vi "DM check burst group.vi"(11 "group":string) -> (3 "String":string)   [LabVIEW 2019, in "DataManagment.lvlib"]
uses:
  DataManagment.lvlib
  SubVIs/Shared/System GV.vi
  SubVIs/Shared/Shared.lvlib
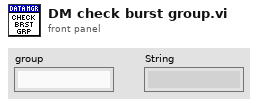
[diagram p1: front panel]
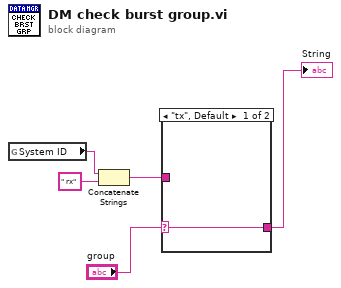
[diagram p0: block diagram]
diagram:
  n1 = global read "System GV.vi" "System ID"() -> (w1:string)
  n2 = Concatenate Strings(w1, " rx" ("group")) -> (w4:string)
  n3 = case shown="\"tx\", Default" "group" {
    selector: "group" -> [w6 _]
    tunnel: w4 -> [_ w7]
    tunnel: [w6 w7] -> w5
    frame "tx", Default {
    }
    frame "rx" {
    }
  }
  "String" <- w5
